vi "pluse frequency_mso7014b_init.vi"(8 "VISA resource name":refnum<visa-resource-name>="tcpip0::192.168.40.220::instr", 11 "Timebase (20.0E-9)":dbl=0.004 format="%#_13g") -> (0 "dt":dbl, 1 "error out":errorcluster, 2 "VISA resource name out":refnum<visa-resource-name>)   [LabVIEW 2016]
uses:
  <instrlib>/Agilent 6000 Series/Public/Configure/Configure Edge Trigger Source.vi
  <instrlib>/Agilent 6000 Series/Agilent 6000 Series.lvlib
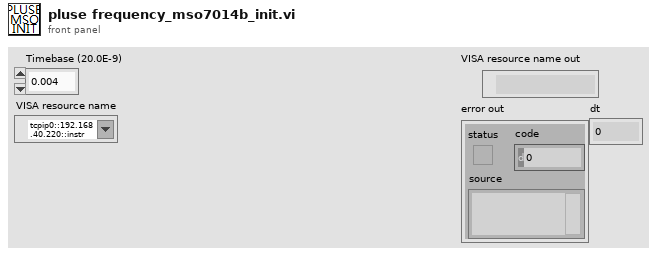
[diagram p1: front panel]
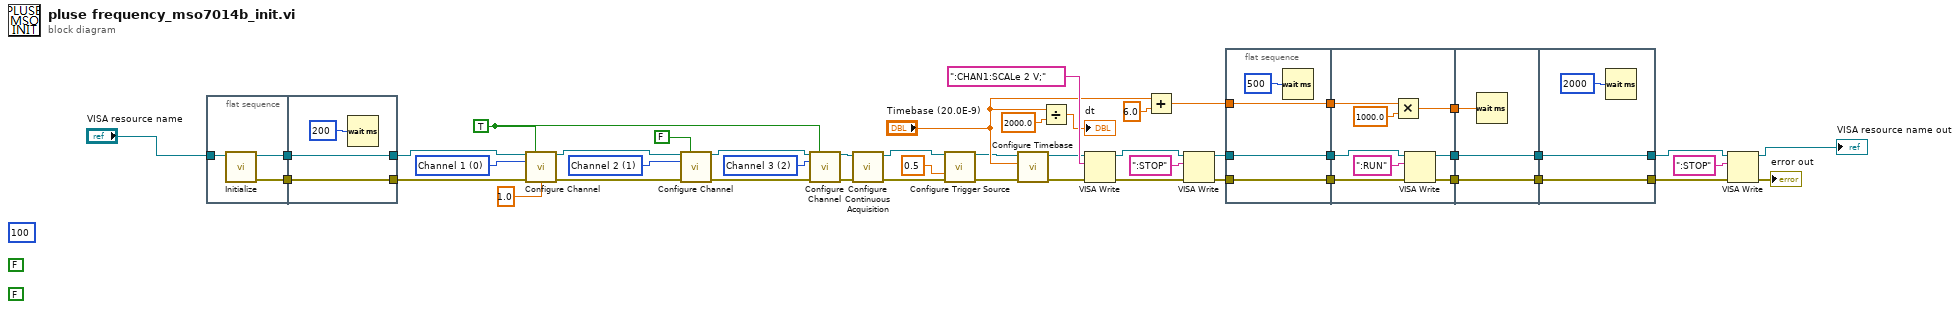
[diagram p0: block diagram]
diagram:
  (unwired) FALSE ("Continuous Acquisition Mode (T: Enable)")
  (unwired) FALSE ("Continuous Acquisition Mode (T: Enable)")
  (unwired) u32 100 ("字节总数")
  w37 = u16 0 items=["Channel 1", "Channel 2", "Channel 3", "Channel 4"] ("Channel (0: Channel 1)")
  w40 = TRUE ("Enable Channel (T: Enable)")
  w43 = u16 2 items=["Channel 1", "Channel 2", "Channel 3", "Channel 4"] ("Channel (0: Channel 1)")
  w45 = u16 1 items=["Channel 1", "Channel 2", "Channel 3", "Channel 4"] ("Channel (0: Channel 1)")
  n1 = flat-sequence {
    tunnel: "VISA resource name" -> [w51]
    tunnel: [w50] -> w21
    tunnel: [w49] -> w20
    tunnel: [w53] -> w38
    tunnel: [w54] -> w39
    tunnel: w21 -> [w54]
    tunnel: w20 -> [w53]
    frame #0 {
      n2 = call <instrlib>:"Initialize.vi"("VISA resource name"=w51) -> ("error out"=w49:errorcluster, "VISA resource name out"=w50:refnum<visa-resource-name>)  [unwired: 9 in]
    }
    frame #1 {
      n3 = Wait (ms)(milliseconds to wait=u32 200 ("等待时间（毫秒）")) -> ()  [unwired: 1 out]
    }
  }
  n4 = call <instrlib>:"Configure Channel.vi"("VISA resource name"=w39, "Enable Channel (T: Enable)"=w40, "Channel (0: Channel 1)"=w37, "error in (no error)"=w38, "Vertical Offset (0.0 V)"=1.0) -> ("VISA resource name out"=w47:refnum<visa-resource-name>, "error out"=w42:errorcluster)  [unwired: 9 in]
  n5 = call <instrlib>:"Configure Channel.vi"("VISA resource name"=w47, "Enable Channel (T: Enable)"=FALSE, "Channel (0: Channel 1)"=w45, "error in (no error)"=w42) -> ("VISA resource name out"=w46:refnum<visa-resource-name>, "error out"=w41:errorcluster)  [unwired: 10 in]
  n6 = call <instrlib>:"Configure Channel.vi"("VISA resource name"=w46, "Enable Channel (T: Enable)"=w40, "Channel (0: Channel 1)"=w43, "error in (no error)"=w41) -> ("VISA resource name out"=w10:refnum<visa-resource-name>, "error out"=w9:errorcluster)  [unwired: 10 in]
  n7 = call <instrlib>:"Configure Continuous Acquisition.vi"("error in (no error)"=w9, "VISA resource name"=w10) -> ("error out"=w3:errorcluster, "VISA resource name out"=w5:refnum<visa-resource-name>)  [unwired: 8 in]
  n8 = call-poly <instrlib>:"Configure Trigger Source.vi"("VISA resource name"=w5, "Trigger Level (0.0 V)"=0.5, "error in (no error)"=w3) -> ("VISA resource name out"=w2:refnum<visa-resource-name>, "error out"=w1:errorcluster)  [unwired: 11 in]
  n9 = call <instrlib>:"Configure Timebase.vi"("error in (no error)"=w1, "Timebase (20.0E-9)"="Timebase (20.0E-9)", "VISA resource name"=w2) -> ("error out"=w33:errorcluster, "VISA resource name out"=w34:refnum<visa-resource-name>)  [unwired: 7 in]
  n10 = Divide(x="Timebase (20.0E-9)", y=2000.0) -> (x/y=→"dt":dbl)
  n11 = VISA Write(VISA resource name=w34, write buffer=":CHAN1:SCALe 2 V;" ("写入缓冲区"), error in (no error)=w33) -> (VISA resource name out=w29:refnum<visa-resource-name>, error out=w27:errorcluster)  [unwired: 1 out]
  n12 = Add(x="Timebase (20.0E-9)", y=6.0) -> (x+y=w6:dbl)
  n13 = VISA Write(VISA resource name=w29, write buffer=":STOP" ("写入缓冲区"), error in (no error)=w27) -> (VISA resource name out=w28:refnum<visa-resource-name>, error out=w26:errorcluster)  [unwired: 1 out]
  n14 = flat-sequence {
    tunnel: w28 -> [w58]
    tunnel: w26 -> [w57]
    tunnel: w6 -> [w55]
    tunnel: [w58] -> w18
    tunnel: [w57] -> w17
    tunnel: [w55] -> w11
    tunnel: [w66] -> w16
    tunnel: [w65] -> w14
    tunnel: w18 -> [w63]
    tunnel: w17 -> [w62]
    tunnel: [w59] -> w12
    tunnel: w11 -> [w61]
    tunnel: w16 -> [w69]
    tunnel: [w69] -> w15
    tunnel: w14 -> [w68]
    tunnel: [w68] -> w13
    tunnel: w12 -> [w67]
    tunnel: [w71] -> w30
    tunnel: [w72] -> w31
    tunnel: w15 -> [w72]
    tunnel: w13 -> [w71]
    frame #0 {
      n15 = Wait (ms)(milliseconds to wait=u32 500 ("等待时间（毫秒）")) -> ()  [unwired: 1 out]
    }
    frame #1 {
      n16 = Multiply(x=w61, y=1000.0) -> (x*y=w59:dbl)
      n17 = VISA Write(VISA resource name=w63, write buffer=":RUN" ("写入缓冲区"), error in (no error)=w62) -> (VISA resource name out=w66:refnum<visa-resource-name>, error out=w65:errorcluster)  [unwired: 1 out]
    }
    frame #2 {
      n18 = Wait (ms)(milliseconds to wait=w67) -> ()  [unwired: 1 out]
    }
    frame #3 {
      n19 = Wait (ms)(milliseconds to wait=u32 2000 ("等待时间（毫秒）")) -> ()  [unwired: 1 out]
    }
  }
  n20 = VISA Write(VISA resource name=w31, write buffer=":STOP" ("写入缓冲区"), error in (no error)=w30) -> (VISA resource name out=→"VISA resource name out":refnum<visa-resource-name>, error out=→"error out":errorcluster)  [unwired: 1 out]
